vi "Ch_data_title_pattern (SubVI).vi"(9 "Единица измерений":string) -> (0 "error out":errorcluster, 2 "Path":path, 3 "Byte Stream File out":refnum<file>)   [LabVIEW 2015]
panel:
  in  "error in":errorcluster
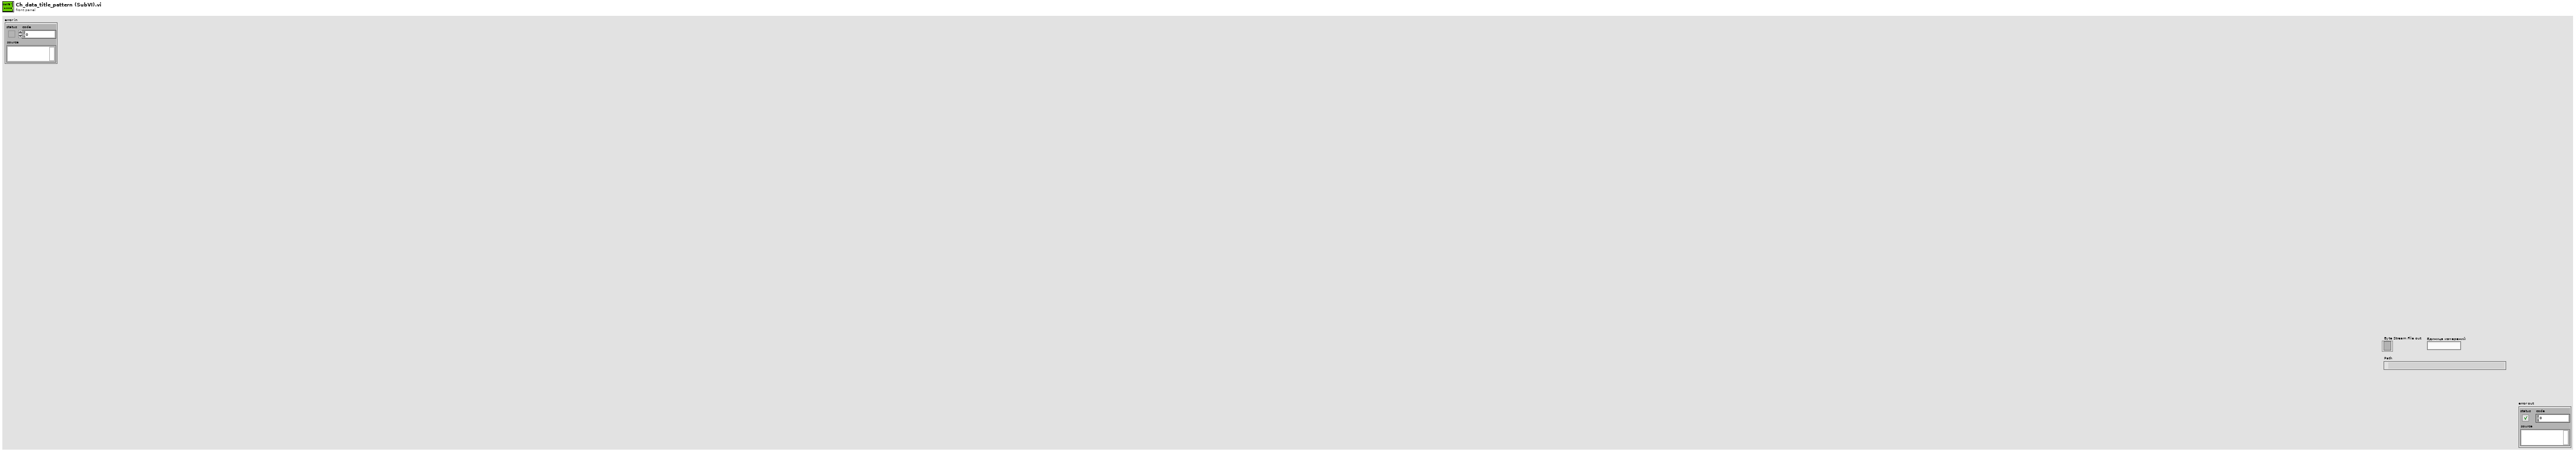
[diagram p1: front panel]
types:
  T1 = enum16{"open", "replace", "create", "open or create", "replace or create", "replace or create with confirmation"}
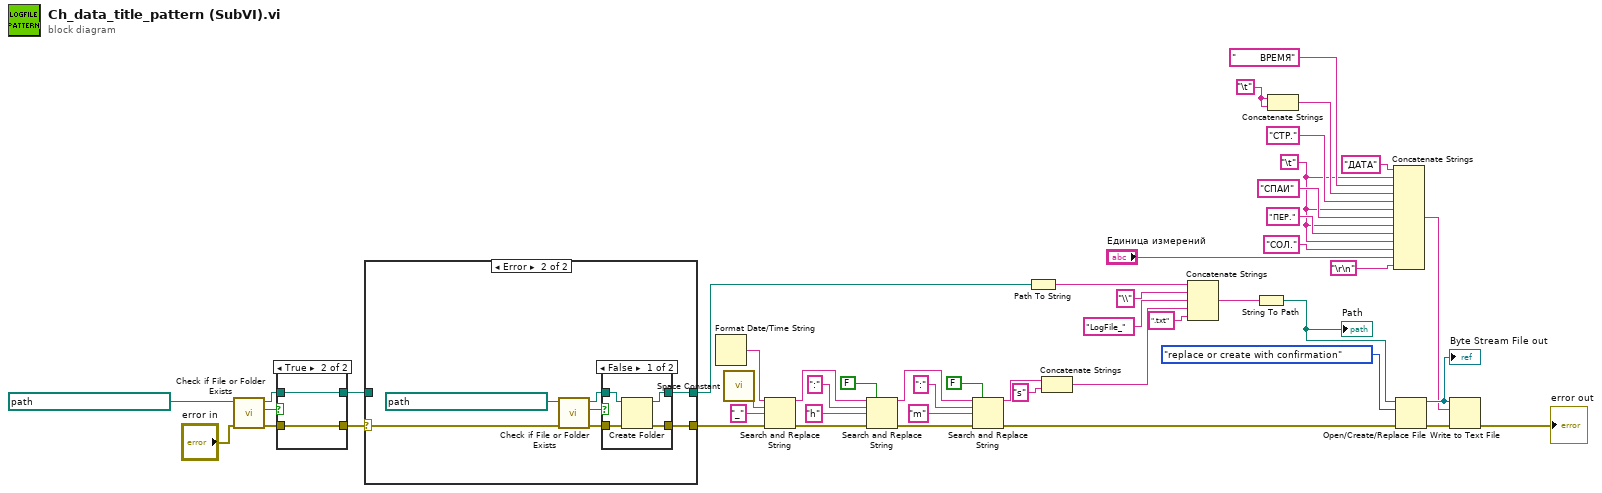
[diagram p0: block diagram]
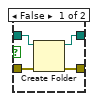
[diagram p4: hidden frame]
diagram:
  w36 = "\t"
  w35 = "\t"
  n1 = call <vilib>:"Check if File or Folder Exists.vi"("error in (no error)"="error in", "path"=path "D:/Лог-файл термометрии" ("path (use dialog)")) -> ("error out"=w31:errorcluster, "file or folder exists?"=w29:bool, "dup path"=w32:path)  [unwired: 7 out]
  n2 = case shown="True" w29 {
    tunnel: [w52 w54] -> w27
    tunnel: w32 -> [w51 w54]
    tunnel: w31 -> [w50 w53]
    tunnel: [w49 w53] -> w28
    frame False {
      n3 = Create Folder(path (use dialog)=w51, error in=w50) -> (created path=w52:path, error out=w49:errorcluster)  [unwired: 2 out]
    }
    frame True {
    }
  }
  n4 = case shown="Error" w28 {
    selector: w28 -> [w55 w57]
    tunnel: w27 -> [w56 _]
    tunnel: [w56 w60] -> w3
    tunnel: [w55 w59] -> w4
    frame No Error {
    }
    frame Error {
      n5 = call <vilib>:"Check if File or Folder Exists.vi"("error in (no error)"=w57, "path"=path "C:/Лог-файл термометрии" ("path (use dialog)")) -> ("error out"=w62:errorcluster, "file or folder exists?"=w61:bool, "dup path"=w63:path)  [unwired: 7 out]
      n6 = case shown="False" w61 {
        tunnel: [w67 w69] -> w60
        tunnel: w63 -> [w66 w69]
        tunnel: w62 -> [w65 w68]
        tunnel: [w64 w68] -> w59
        frame False {
          n7 = Create Folder(path (use dialog)=w66, error in=w65) -> (created path=w67:path, error out=w64:errorcluster)  [unwired: 2 out]
        }
        frame True {
        }
      }
    }
  }
  n8 = Format Date/Time String() -> (date/time string=w25:string)  [unwired: 3 out]
  n9 = call <vilib>:"Space Constant.vi"() -> ("String"=w6:string)
  n10 = Search and Replace String(input string=w25, search string=w6, replace string="_" ("replace string (\"\")"), error in=w4) -> (result string=w8:string, error out=w18:errorcluster)  [unwired: 6 out]
  n11 = Search and Replace String(replace all?=FALSE ("replace all? (F)"), input string=w8, search string=":", replace string="h" ("replace string (\"\")"), error in=w18) -> (result string=w15:string, error out=w19:errorcluster)  [unwired: 5 out]
  n12 = Search and Replace String(replace all?=FALSE ("replace all? (F)"), input string=w15, search string=":", replace string="m" ("replace string (\"\")"), error in=w19) -> (result string=w20:string, error out=w2:errorcluster)  [unwired: 5 out]
  n13 = Path To String(path=w3) -> (string=w16:string)
  n14 = Concatenate Strings(w20, "s" ("string")) -> (w23:string)
  n15 = Concatenate Strings(w16, "\\" ("string"), "LogFile_" ("string"), w23, ".txt" ("default name")) -> (w5:string)
  n16 = String To Path(string=w5) -> (path=w1:path)
  "Path" <- w1
  n17 = Concatenate Strings(w36, w36) -> (w37:string)
  n18 = Concatenate Strings("ДАТА" ("string"), w35, "        ВРЕМЯ" ("string"), w37, "СТР." ("string"), w35, "СПАИ" ("string"), w35, "ПЕР." ("string"), w35, "СОЛ." ("string"), "Единица измерений", "\r\n") -> (w39:string)
  n19 = Open/Create/Replace File(file path (use dialog)=w1, error in=w2, operation (0:open)=T1."replace or create with confirmation") -> (refnum out=w42:refnum<file>, error out=w40:errorcluster)  [unwired: 4 out]
  "Byte Stream File out" <- w42
  n20 = Write to Text File(file (use dialog)=w42, text=w39, error in=w40) -> (error out=→"error out":errorcluster)  [unwired: 3 out]
